vi "HB_CheckChecksum.vi"(11 "String":string) -> (2 "Checksum Received":string, 3 "Checksum Matches":bool)   [LabVIEW 2016]
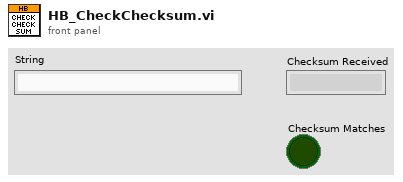
[diagram p1: front panel]
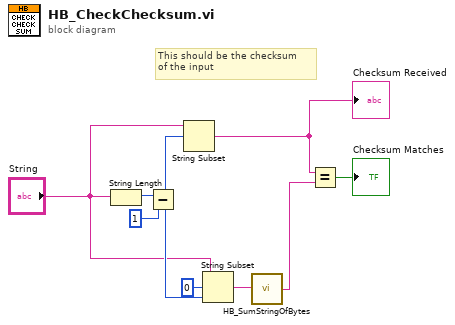
[diagram p0: block diagram]
diagram:
  # "This should be the checksum \nof the input"
  n1 = String Length(string="String") -> (length=w9:i32)
  n2 = Subtract(x=w9, y=1) -> (x-y=w5:i32)
  n3 = String Subset(string="String", offset (0)=w5) -> (substring=w7:string)  [unwired: 1 in]
  "Checksum Received" <- w7
  n4 = String Subset(string="String", offset (0)=0, length (rest)=w5) -> (substring=w2:string)
  n5 = call "HB_SumStringOfBytes.vi"("String Of Bytes"=w2) -> ("Sum as String"=w1:string)
  n6 = Equal?(x=w7, y=w1) -> (x = y?=→"Checksum Matches":bool)
